vi "Grap Image_teststand.vi"(0 "Refnum in":T2, 4 "Trigger is on ?":bool=TRUE, 5 "error in":errorcluster) -> (14 "Refnum out":T2, 16 "Pass?":bool, 19 "error out":errorcluster)   [LabVIEW 2015]
uses:
  <vilib>/userdefined/High Color/IMAQdx.ctl
  <vilib>/vision/driver/NI_Vision_Acquisition_Software.lvlib
panel:
  in  "Exit":bool
  out "Process Image":T1(plugin-control)
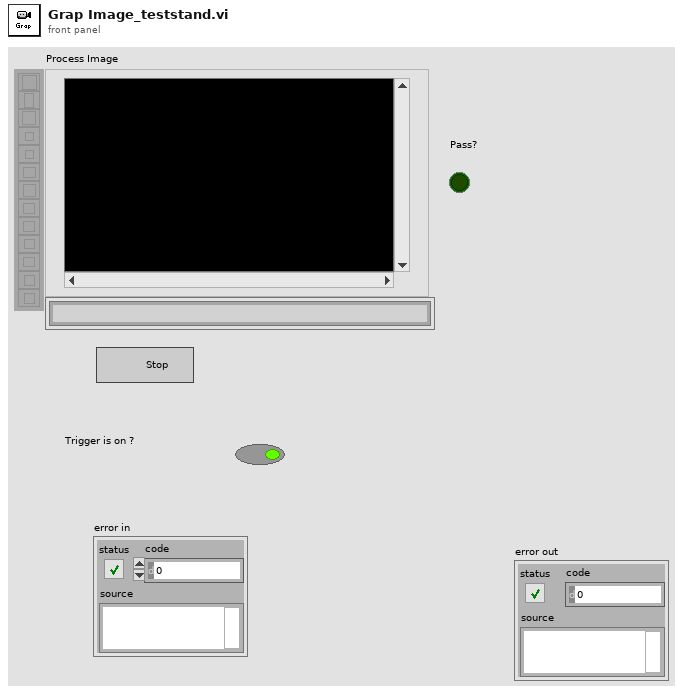
[diagram p1: front panel]
types:
  T1 = typedef "IMAQ Image.ctl" = refnum<image>
  T2 = typedef "IMAQdx.ctl" = refnum<k21>
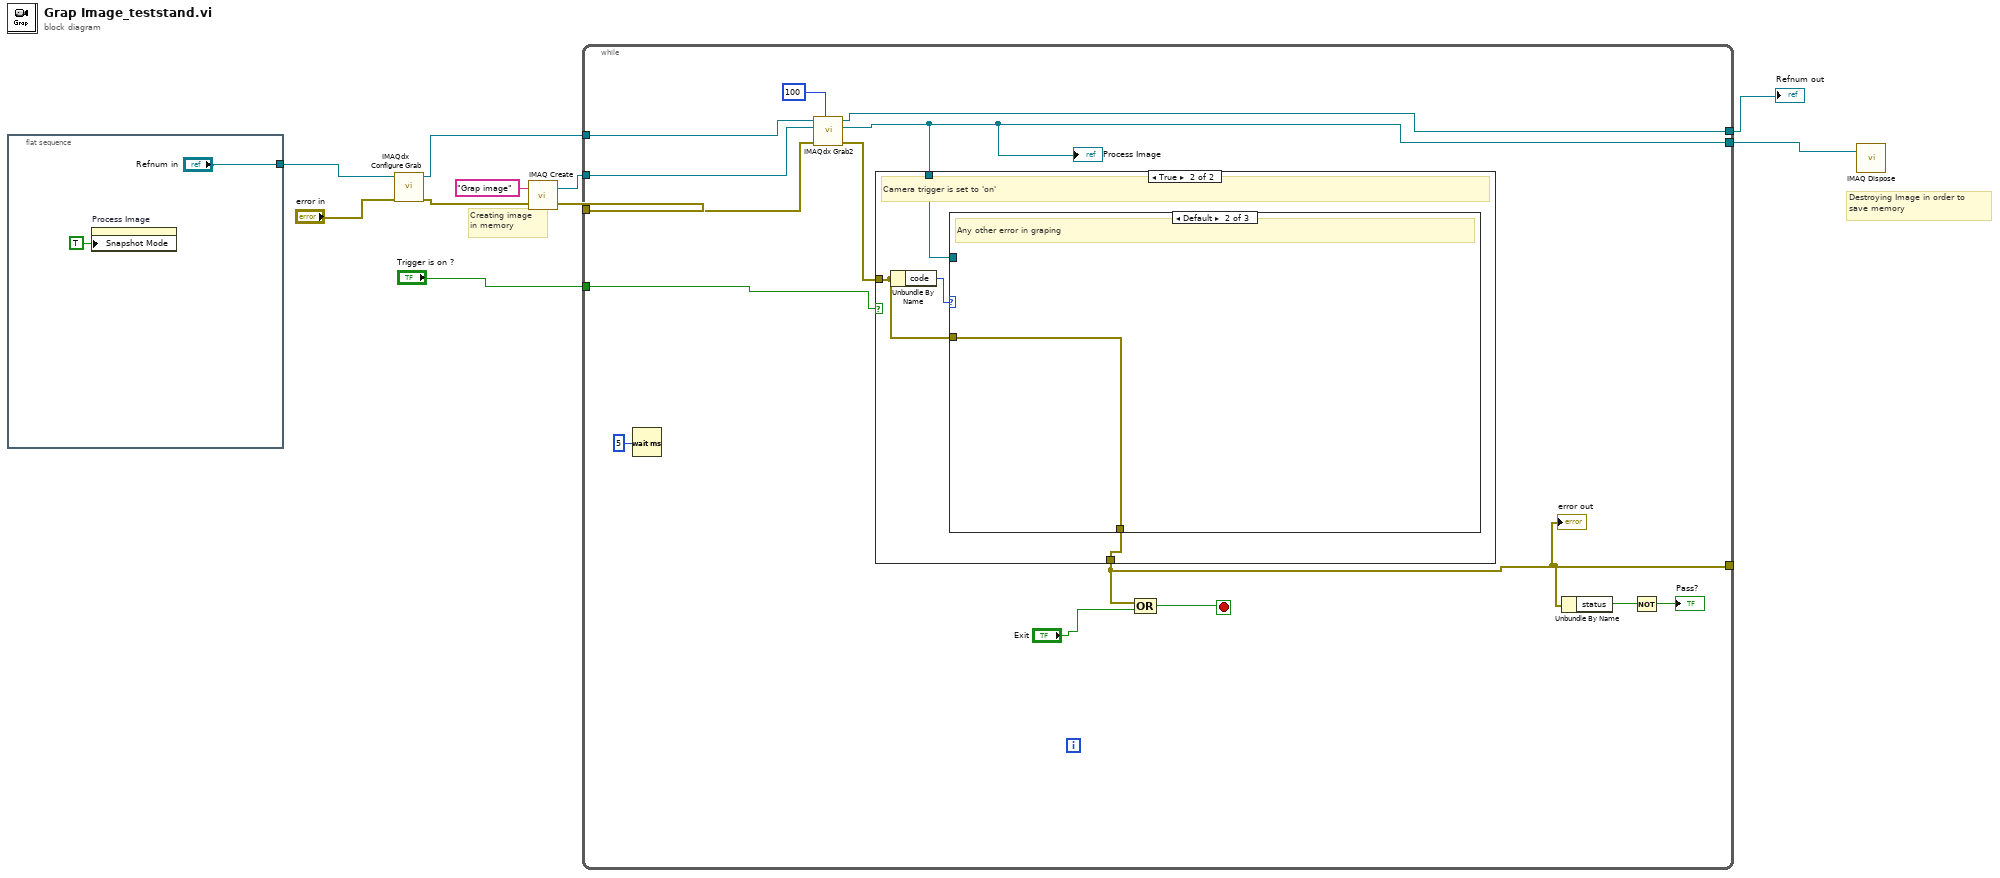
[diagram p0: block diagram]
diagram:
  # "Destroying Image in order to\nsave memory"
  # "Creating image\nin memory"
  n1 = flat-sequence {
    tunnel: ["Refnum in"] -> w2
    frame #0 {
      n2 = property on="Process Image" class="ImageControl"("Snapshot Mode"=TRUE) -> ()  [unwired: 2 in, 2 out]
    }
  }
  n3 = call <vilib>:"IMAQdx Configure Grab.vi"("error in"="error in", "Session In"=w2) -> ("error out"=w9:errorcluster, "Session Out"=w5:T2)  [unwired: 8 in]
  n4 = call "IMAQ Create"("Image Name"="Grap image", "error in (no error)"=w9) -> ("New Image"=w7:T1, "error out"=w10:errorcluster)  [unwired: 3 in]
  n5 = while {
    tunnel: w5 -> [w26]
    tunnel: w7 -> [w25]
    tunnel: [w18] -> w8
    tunnel: w10 -> [w24]
    tunnel: [w22] -> w4
    tunnel: [w15] -> _
    tunnel: "Trigger is on ?" -> [w20]
    stop <- w23 stop-if-true
    n6 = Wait (ms)(milliseconds to wait=u32 5) -> ()  [unwired: 1 out]
    n7 = call <vilib>:"IMAQdx Grab2.vi"("Timeout (ms)"=100, "error in"=w24, "Image In"=w25, "Session In"=w26) -> ("error out"=w19:errorcluster, "Image Out"=w18:T1, "Session Out"=w22:T2)  [unwired: 4 in, 1 out]
    "Process Image" <- w18
    n8 = case shown="True" w20 {
      tunnel: w18 -> [_ w30]
      tunnel: w19 -> [w27 w29]
      tunnel: [w27 w28] -> w15
      frame False {
        # "Camera trigger is set to 'off'"
      }
      frame True {
        # "Camera trigger is set to 'on'"
        n9 = Unbundle By Name(w29) -> ("code"=w31:i32)
        n10 = case shown="Default" w31 {
          tunnel: w30 -> [_ _ _]
          tunnel: w29 -> [_ w32 _]
          tunnel: [_ w32 _] -> w28
          frame 0 {
            # "No error"
          }
          frame Default {
            # "Any other error in graping"
          }
          frame -1074360293 {
            # "Time out error\nhas to be ignored \nto wait for trigger"
          }
        }
      }
    }
    "error out" <- w15
    n11 = Compound Arithmetic op=OR(w15, "Exit") -> (w23:bool)
    n12 = Unbundle By Name(w15) -> ("status"=w16:bool)
    n13 = Not(x=w16) -> (.not. x?=→"Pass?":bool)
  }
  "Refnum out" <- w4
  n14 = call "IMAQ Dispose"("Image"=w8) -> ()  [unwired: 5 in, 1 out]
